vi "JKI SM Editor - VIPC File -- List Packages__vipm_api_vipm_api.vi"(8 "error in (no error)":errorcluster, 11 "VIPC File Path":path) -> (0 "error out":errorcluster, 1 "VIPC LabVIEW Version":string, 2 "Package List":string[](array[string]), 3 "VIPC File Path (dup)":path)   [LabVIEW 2013]
doc: "Copyright 2009-2012 JKI"
uses:
  <vilib>/JKI/_VIPM API_internal_deps/ZLIB Open Unzip Archive__ogtk16290F98F102B0FBD386C52BCC276B65.vi
  <vilib>/JKI/_VIPM API_internal_deps/ZLIB Extract Stream__ogtk16290F98F102B0FBD386C52BCC276B65.vi
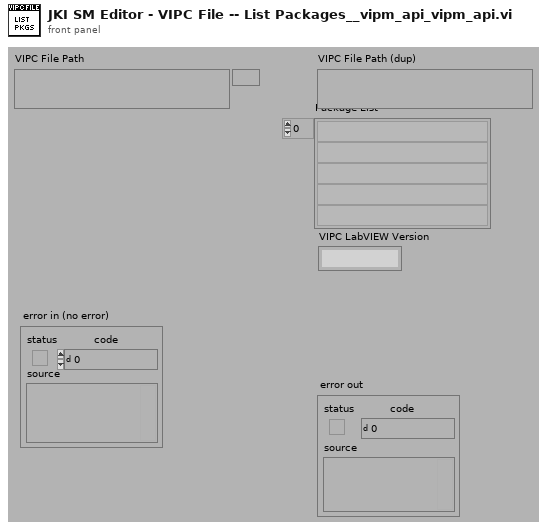
[diagram p1: front panel]
types:
  T1 = typedef "ZLIB Unzip Handle__ogtk16290F98F102B0FBD386C52BCC276B65.ctl" = refnum<k1>
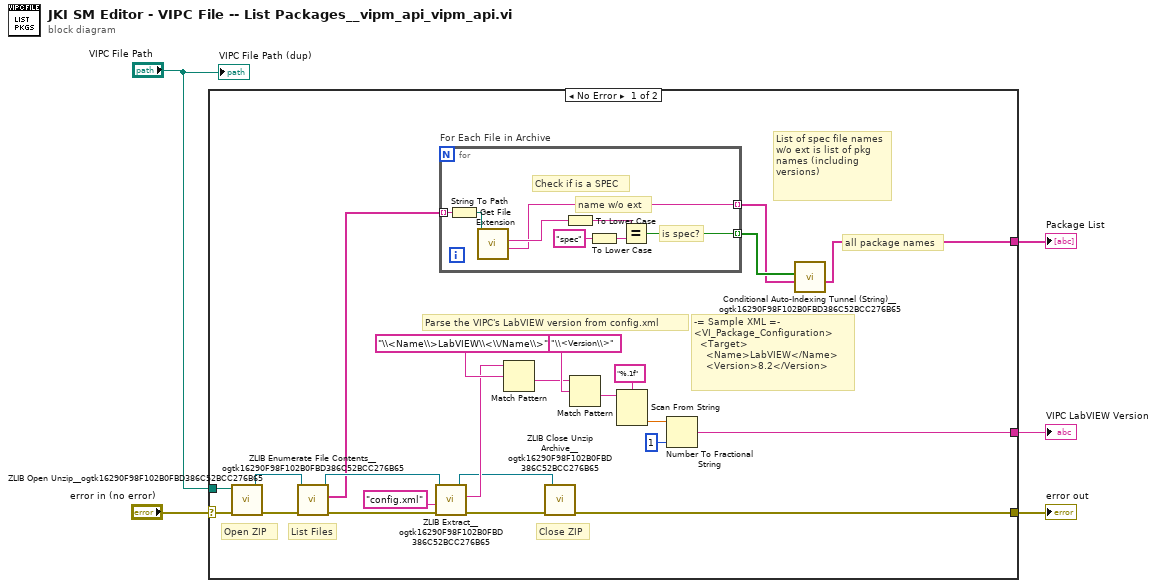
[diagram p0: block diagram]
diagram:
  n1 = case shown="No Error" "error in (no error)" {
    selector: "error in (no error)" -> [w25 w37]
    tunnel: [w6 _] -> w4
    tunnel: [w9 w37] -> w3
    tunnel: "VIPC File Path" -> [w26 _]
    tunnel: [w16 _] -> w1
    frame No Error {
      # "all package names"
      # "-= Sample XML =-\n<VI_Package_Configuration>\n  <Target>\n    <Name>LabVIEW</Name>\n    <Version>8.2</Version>"
      # "Parse the VIPC's LabVIEW version from config.xml"
      # "Close ZIP"
      # "List Files"
      # "Open ZIP"
      # "List of spec file names w/o ext is list of pkg names (including versions)"
      n2 = call-poly <vilib>:"ZLIB Open Unzip__ogtk16290F98F102B0FBD386C52BCC276B65.vi"("error in (no error)"=w25, "archive name"=w26) -> ("error out"=w28:errorcluster, "unzip Refnum"=w27:T1)  [unwired: 4 in]
      n3 = call <vilib>:"ZLIB Enumerate File Contents__ogtk16290F98F102B0FBD386C52BCC276B65.vi"("error in (no error)"=w28, "unzip Refnum"=w27) -> ("error out"=w13:errorcluster, "file names"=w12:string[], "unzip Refnum out"=w24:T1)  [unwired: 5 in, 2 out]
      n4 = call-poly <vilib>:"ZLIB Extract__ogtk16290F98F102B0FBD386C52BCC276B65.vi"("error in (no error)"=w13, "internal name"="config.xml" ("extension"), "unzip Refnum"=w24) -> ("error out"=w10:errorcluster, "byte stream"=w14:string, "unzip Refnum out"=w11:T1)  [unwired: 4 in]
      n5 = for "For Each File in Archive" {
        tunnel: w12 -> [w32] mode=indexing
        tunnel: [w33] -> w8 mode=indexing
        tunnel: [w30] -> w7 mode=indexing
        # "is spec?"
        # "name w/o ext"
        # "Check if is a SPEC"
        n6 = String To Path(string=w32) -> (path=w29:path)
        n7 = call <vilib>:"Get File Extension.vi"("file"=w29) -> ("filename without extension"=w30:string, "lowercase file extension"=w31:string)  [unwired: 7 in, 2 out]
        n8 = To Lower Case(string=w31) -> (all lower case string=w35:string)
        n9 = To Lower Case(string="spec" ("extension")) -> (all lower case string=w34:string)
        n10 = Equal?(x=w35, y=w34) -> (x = y?=w33:bool)
      }
      n11 = Match Pattern(string=w14, regular expression="\\<Name\\>LabVIEW\\<\\/Name\\>") -> (after substring=w21:string)  [unwired: 1 in, 3 out]
      n12 = call <vilib>:"ZLIB Close Unzip Archive__ogtk16290F98F102B0FBD386C52BCC276B65.vi"("error in (no error)"=w10, "unzip Refnum"=w11) -> ("error out"=w9:errorcluster)  [unwired: 5 in]
      n13 = Match Pattern(string=w21, regular expression="\\<Version\\>") -> (after substring=w18:string)  [unwired: 1 in, 3 out]
      n14 = Scan From String(format string="%.1f", input string=w18) -> (output 1=w19:dbl)  [unwired: 3 in, 3 out]
      n15 = Number To Fractional String(number=w19, precision (6)=i16 1) -> (F-format string=w16:string)  [unwired: 2 in]
      n16 = call <vilib>:"Conditional Auto-Indexing Tunnel (String)__ogtk16290F98F102B0FBD386C52BCC276B65.vi"("Array in"=w7, "Elements to keep"=w8) -> ("Filtered Array out"=w6:string[])  [unwired: 5 in]
    }
    frame Error {
    }
  }
  "error out" <- w3
  "Package List" <- w4
  "VIPC LabVIEW Version" <- w1
  "VIPC File Path (dup)" <- "VIPC File Path"
